vi "RS_RTO1024_Error_check.vi"(4 "Driver Name":T8, 6 "Error Code":T7, 8 "error in":T6, 11 "DriverConnect in":T1={"InterfaceType"=enum."VISA", "OpenedSession"="", "InterfaceSettings"={"Interface"=enum."RS232", "EOS 4 read"=enum."LF (\\n)", "EOS 4 write"=enum."LF (\\n)", "TMO, ms"=10000, "Sett"=variant(cluster{"Baud Rate":u32, "Data Bits":u16, "Parity":u16, "Stop Bits":u16, "Flow Control":u16, "Eho":bool} {"Baud Rate"=75, "Data Bits"=0, "Parity"=0, "Stop Bits"=0, "Flow Control"=0, "Eho"=FALSE})}}) -> (0 "error out":T6, 3 "DriverConnect out":T1={"InterfaceType"=enum."VISA", "OpenedSession"="", "InterfaceSettings"={"Interface"=enum."RS232", "EOS 4 read"=enum."LF (\\n)", "EOS 4 write"=enum."LF (\\n)", "TMO, ms"=10000, "Sett"=variant(cluster{"Baud Rate":u32, "Data Bits":u16, "Parity":u16, "Stop Bits":u16, "Flow Control":u16, "Eho":bool} {"Baud Rate"=75, "Data Bits"=0, "Parity"=0, "Stop Bits"=0, "Flow Control"=0, "Eho"=FALSE})}})   [LabVIEW 2018]
uses:
  MOKO_LabViewLibrary/MokoLowLevel/MokoLowLovelControl/MLLC_DriverName.ctl
  MOKO_LabViewLibrary/MokoLowLevel/MokoLowLovelControl/MLLC_ErrorCode.ctl
  MOKO_LabViewLibrary/MokoLowLevel/MokoLowLovelControl/MLLC_Error.ctl
  MOKO_LabViewLibrary/MokoLowLevel/MokoLowLovelControl/MLLC_ConnectCluster.ctl
  MOKO_LabViewLibrary/MokoLowLevel/MokoLowLovelControl/MLLC_InterfaceType.ctl
  MOKO_LabViewLibrary/MokoLowLevel/MokoLowLovelControl/MLLC_OpenedSession.ctl
  MOKO_LabViewLibrary/MokoLowLevel/MokoLowLovelControl/MLLC_InterfaceSettings.ctl
  MOKO_LabViewLibrary/MokoLowLevel/MokoLowLovelControl/MLLC_InterfaceKind.ctl
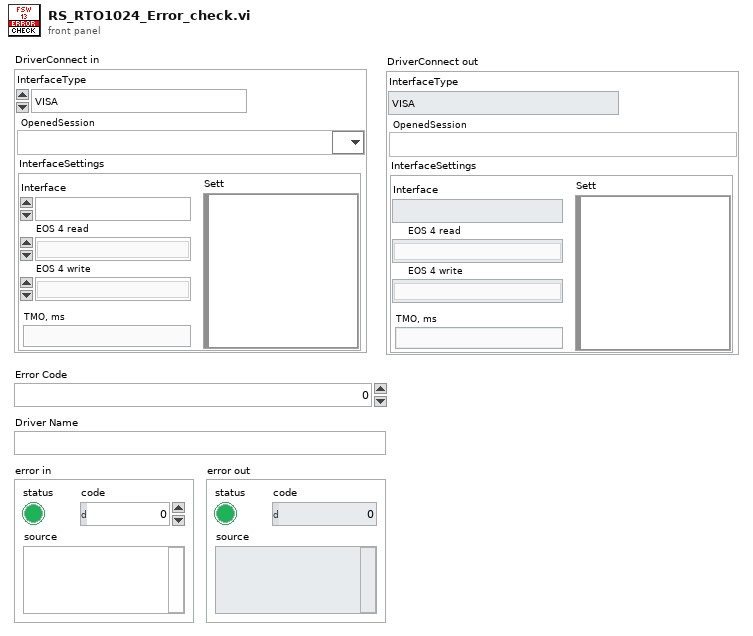
[diagram p1: front panel]
types:
  T1 = typedef "MLLC_ConnectCluster.ctl" = cluster{"InterfaceType":T2, "OpenedSession":T3, "InterfaceSettings":T4}
  T2 = typedef "MLLC_InterfaceType.ctl" = enum16{"VISA", "Prologix USB-GPIB"}
  T3 = typedef "MLLC_OpenedSession.ctl" = refnum<visa-resource-name>
  T4 = typedef "MLLC_InterfaceSettings.ctl" = cluster{"Interface":T5, "EOS 4 read":enum16{"Default (=EOS 4 write)", "CR (\\r)", "LF (\\n)", "None"}, "EOS 4 write":enum16{"CR+LF (\\r\\n)", "CR (\\r)", "LF (\\n)", "None"}, "TMO, ms":i32, "Sett":variant}
  T5 = typedef "MLLC_InterfaceKind.ctl" = enum16{"RS232", "GPIB", "USB", "Ethernet", "another"}
  T6 = typedef "MLLC_Error.ctl" = errorcluster
  T7 = typedef "MLLC_ErrorCode.ctl" = u32
  T8 = typedef "MLLC_DriverName.ctl" = string
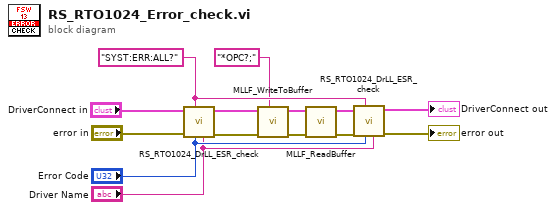
[diagram p0: block diagram]
diagram:
  w11 = "SYST:ERR:ALL?" ("Error Query")
  n1 = call "RS_RTO1024_DrLL_ESR_check.vi"("Driver Name"="Driver Name", "Error Code"="Error Code", "Error Query"=w11, "Error In"="error in", "DriverConnect in"="DriverConnect in") -> ("Error Out"=w8:errorcluster, "DriverConnect out"=w9:T1)  [unwired: 5 in]
  n2 = call "MLLF_WriteToBuffer.vi"("String"="*OPC?;", "error in"=w8, "DriverConnect in"=w9) -> ("error out"=w13:T6, "DriverConnect out"=w12:T1)  [unwired: 5 in]
  n3 = call "MLLF_ReadBuffer.vi"("Error In"=w13, "DriverConnect in"=w12) -> ("Error Out"=w7:errorcluster, "DriverConnect out"=w10:T1)  [unwired: 6 in, 1 out]
  n4 = call "RS_RTO1024_DrLL_ESR_check.vi"("Driver Name"="Driver Name", "Error Code"="Error Code", "Error Query"=w11, "Error In"=w7, "DriverConnect in"=w10) -> ("Error Out"=→"error out":errorcluster, "DriverConnect out"=→"DriverConnect out":T1)  [unwired: 5 in]
